vi "Lasers.vi"(0 "Turn on?":bool, 2 "SRV In":string) -> (4 "SRV Out":string="169.254.0.10")   [LabVIEW 2009]
panel:
  out "Reply":string
  # "This LabVIEW item is deprecated.\n\nIt is believed to be unused and will be removed in a future version of SRV."
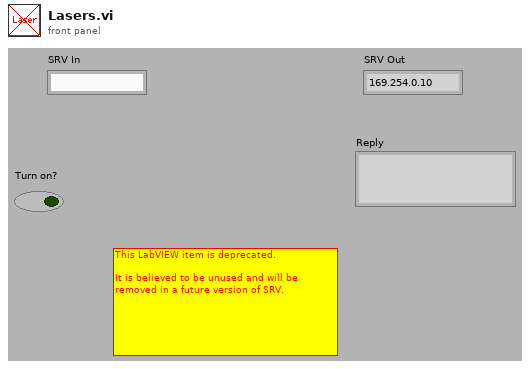
[diagram p1: front panel]
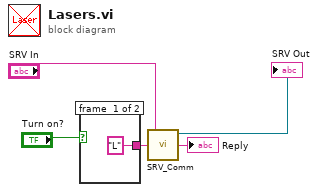
[diagram p0: block diagram]
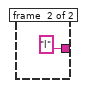
[diagram p2: hidden frame]
diagram:
  n1 = case shown="True" "Turn on?" {
    tunnel: ["L" ("Command Sent") "l" ("Command Sent")] -> w3
    frame #0 {
    }
    frame #1 {
    }
  }
  n2 = call "SRV_Comm.vi"("Command Sent"=w3, "SRV In"="SRV In") -> ("Reply"=→"Reply":string, "SRV Out"=→"SRV Out":refnum<k5>)  [unwired: 1 in, 1 out]
